vi "ni579x Send FAM Register Operations.vi"(0 "Register Bus":refnum<class "ni579x Register Bus v1 Host.lvclass">=refnum, 1 "scope":string, 5 "FAM Register Operations":T1[](array[typedef]) {"Write Data" format="%x"; "Address" format="%06x"; "FAM Register Offset" items=["ADC"=1, "DAC"=2, "Clock Distribution Chip"=3, "Frequency/Phase Adjust DAC"=4, "EEPROM"=5, "EEPROM Commands"=6, "LO1"=7, "Rx Atten Pre-LNA"=9, "Rx Atten Post-LNA"=10, "Tx Atten"=11]}, 11 "Error In":errorcluster) -> (4 "Register Bus (out)":refnum<class "ni579x Register Bus v1 Host.lvclass">, 6 "FAM Register Read Data":u32[](array[numeric]) format="%.0x", 15 "Error Out":errorcluster)   [LabVIEW 2013]
uses:
  <instrlib>/ni579x/Register Bus/v1/Host/ni579x Register Bus v1 Host.lvclass
  <instrlib>/ni579x/Config/v1/Shared/Types/ni579x FAM Register Operation.ctl
  <instrlib>/ni579x/Config/v1/Shared/Types/ni579x FAM Register Offset.ctl
  <instrlib>/ni579x/Config/v1/Shared/Types/ni579x Register Bus Subsystem ID.ctl
  <instrlib>/ni579x/Register Bus/v1/Host/Public/Register Write.ctl
  <instrlib>/ni579x/Register Bus/v1/Host/Public/Register Read Request.ctl
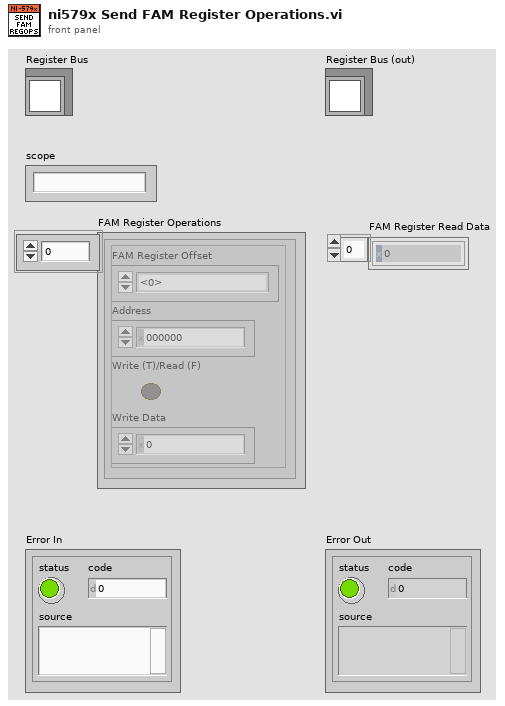
[diagram p1: front panel]
types:
  T1 = typedef "ni579x FAM Register Operation.ctl" = cluster{"FAM Register Offset":T2, "Address":u32, "Write (T)/Read (F)":bool, "Write Data":u32}
  T2 = typedef "ni579x FAM Register Offset.ctl" = u8
  T3 = typedef "ni579x Register Bus v1 Host.lvclass/Register Write.ctl" = cluster{"subsystem":u8, "address":u16, "data":u32}
  T4 = typedef "ni579x Register Bus v1 Host.lvclass/Register Read Request.ctl" = cluster{"subsystem":u8, "address":u16}
  T5 = typedef "ni579x Register Bus Subsystem ID.ctl" = u8
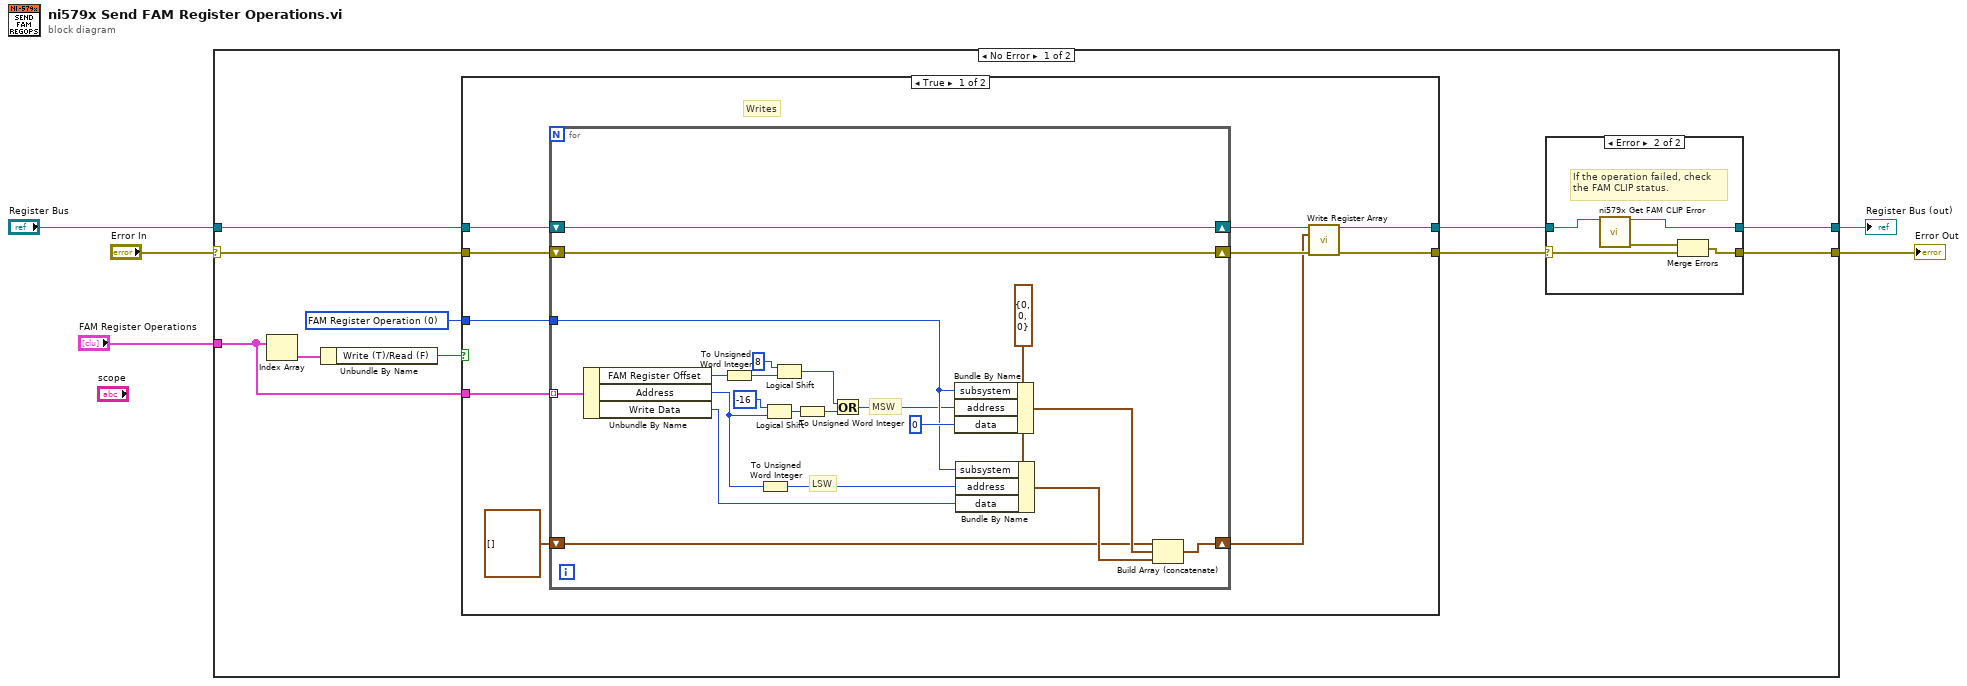
[diagram p0: block diagram]
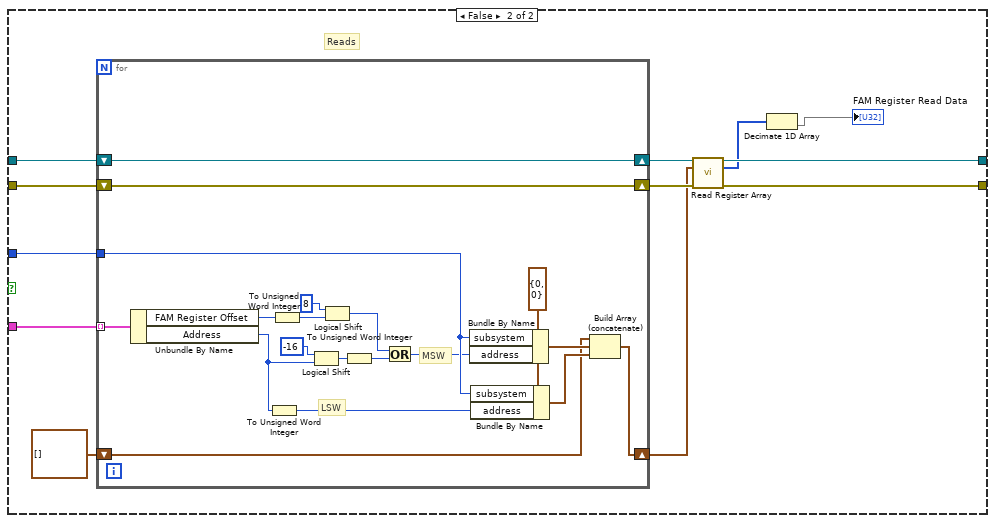
[diagram p3: hidden frame]
diagram:
  n1 = case shown="No Error" "Error In" {
    selector: "Error In" -> [w12 w86]
    tunnel: [w7 w86] -> w4
    tunnel: "Register Bus" -> [w11 w85]
    tunnel: "FAM Register Operations" -> [w15 _]
    tunnel: [w8 w85] -> w2
    frame No Error {
      w6 = T5 0 items=["FAM Register Operation"=0, "User Command"=16, "Synchronization"=32] ("Subsystem ID")
      n2 = Index Array(array=w15) -> (element=w14:T1)  [unwired: 1 in]
      n3 = Unbundle By Name(w14) -> ("Write (T)/Read (F)"=w13:bool)
      n4 = case shown="True" w13 {
        tunnel: w15 -> [w32 w65]
        tunnel: w12 -> [w31 w64]
        tunnel: w11 -> [w30 w63]
        tunnel: [w25 w60] -> w9
        tunnel: [w24 w59] -> w10
        tunnel: w6 -> [w29 w57]
        frame True {
          # "Writes"
          n5 = for {
            tunnel: w32 -> [w53] mode=indexing
            shift-right: [w33] -> w26
            shift-left: w31 -> [w33]
            shift-right: [w34] -> w27
            shift-left: w30 -> [w34]
            tunnel: w29 -> [w45]
            shift-right: [w36] -> w23
            shift-left: T3[] [] -> [w35]
            w46 = T3 {"subsystem"=0, "address"=0, "data"=0} ("register write")
            # "LSW"
            # "MSW"
            n6 = Unbundle By Name(w53) -> ("FAM Register Offset"=w44:T2, "Address"=w48:u32, "Write Data"=w52:u32)
            n7 = To Unsigned Word Integer(number=w44) -> (unsigned 16bit integer=w43:u16)
            n8 = To Unsigned Word Integer(number=w48) -> (unsigned 16bit integer=w47:u16)
            n9 = Logical Shift(y=i8 -16, x=w48) -> (x << y=w49:u32)
            n10 = Logical Shift(y=i8 8, x=w43) -> (x << y=w41:u16)
            n11 = To Unsigned Word Integer(number=w49) -> (unsigned 16bit integer=w40:u16)
            n12 = Or(x=w41, y=w40) -> (x .or. y?=w39:u16)
            n13 = Bundle By Name(cluster=w46, "subsystem"=w45, "address"=w39, "data"=u32 0) -> (w37:T3)
            n14 = Bundle By Name(cluster=w46, "subsystem"=w45, "address"=w47, "data"=w52) -> (w38:T3)
            n15 = Build Array (concatenate)(w35, w37, w38) -> (w36:T3[])
          }
          n16 = call <instrlib>:"Write Register Array.vi"("session in"=w27, "register writes"=w23, "error in"=w26) -> ("session out"=w25:refnum<class "ni579x Register Bus v1 Host.lvclass">, "error out"=w24:errorcluster)  [unwired: 11 in]
        }
        frame False {
          # "Reads"
          n17 = for {
            tunnel: w65 -> [w84] mode=indexing
            shift-right: [w83] -> w62
            shift-left: w64 -> [w83]
            shift-right: [w82] -> w61
            shift-left: w63 -> [w82]
            tunnel: w57 -> [w72]
            shift-right: [w74] -> w56
            shift-left: T4[] [] -> [w73]
            w79 = T4 {"subsystem"=0, "address"=0} ("register read request")
            # "LSW"
            # "MSW"
            n18 = Unbundle By Name(w84) -> ("FAM Register Offset"=w69:T2, "Address"=w78:u32)
            n19 = To Unsigned Word Integer(number=w78) -> (unsigned 16bit integer=w77:u16)
            n20 = To Unsigned Word Integer(number=w69) -> (unsigned 16bit integer=w71:u16)
            n21 = Logical Shift(y=i8 -16, x=w78) -> (x << y=w80:u32)
            n22 = Logical Shift(y=i8 8, x=w71) -> (x << y=w67:u16)
            n23 = To Unsigned Word Integer(number=w80) -> (unsigned 16bit integer=w68:u16)
            n24 = Or(x=w67, y=w68) -> (x .or. y?=w66:u16)
            n25 = Bundle By Name(cluster=w79, "subsystem"=w72, "address"=w66) -> (w76:T4)
            n26 = Bundle By Name(cluster=w79, "subsystem"=w72, "address"=w77) -> (w75:T4)
            n27 = Build Array (concatenate)(w73, w76, w75) -> (w74:T4[])
          }
          n28 = call <instrlib>:"Read Register Array.vi"("session in"=w61, "register read requests"=w56, "error in"=w62) -> ("session out"=w60:refnum<class "ni579x Register Bus v1 Host.lvclass">, "data"=w58:u32[], "error out"=w59:errorcluster)  [unwired: 10 in]
          n29 = Decimate 1D Array(w58) -> (→"FAM Register Read Data":u32[])  [unwired: 1 out]
        }
      }
      n30 = case shown="Error" w10 {
        selector: w10 -> [w16 w22]
        tunnel: w9 -> [w17 w21]
        tunnel: [w17 w18] -> w8
        tunnel: [w16 w19] -> w7
        frame No Error {
        }
        frame Error {
          # "If the operation failed, check \nthe FAM CLIP status."
          n31 = call <instrlib>:"ni579x Get FAM CLIP Error.vi"("Register Bus"=w21) -> ("Register Bus (out)"=w18:refnum<class "ni579x Register Bus v1 Host.lvclass">, "Error Out"=w20:errorcluster)  [unwired: 13 in]
          n32 = Merge Errors(w20, w22) -> (w19:errorcluster)
        }
      }
    }
    frame Error {
    }
  }
  "Error Out" <- w4
  "Register Bus (out)" <- w2
